vi "Adjust Graph.vi"(7 "log?":bool, 8 "error in (no error)":errorcluster, 9 "Secondary Graph":refnum<vi>, 10 "Primary Graph":refnum<vi>, 11 "Scan Driver.lvclass":refnum<class "Scan Driver.lvclass">) -> (0 "error out":errorcluster, 2 "High":dbl, 3 "Scan Driver.lvclass out":refnum<class "Scan Driver.lvclass">)   [LabVIEW 2015, in "Scan Driver.lvclass"]
uses:
  Scan Driver.lvclass
  Scan Driver.lvclass/Scan Driver.ctl
  Scanners/Scanner/Scanner.lvclass
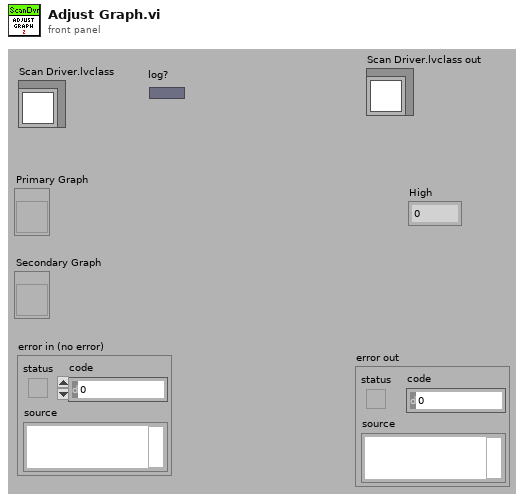
[diagram p1: front panel]
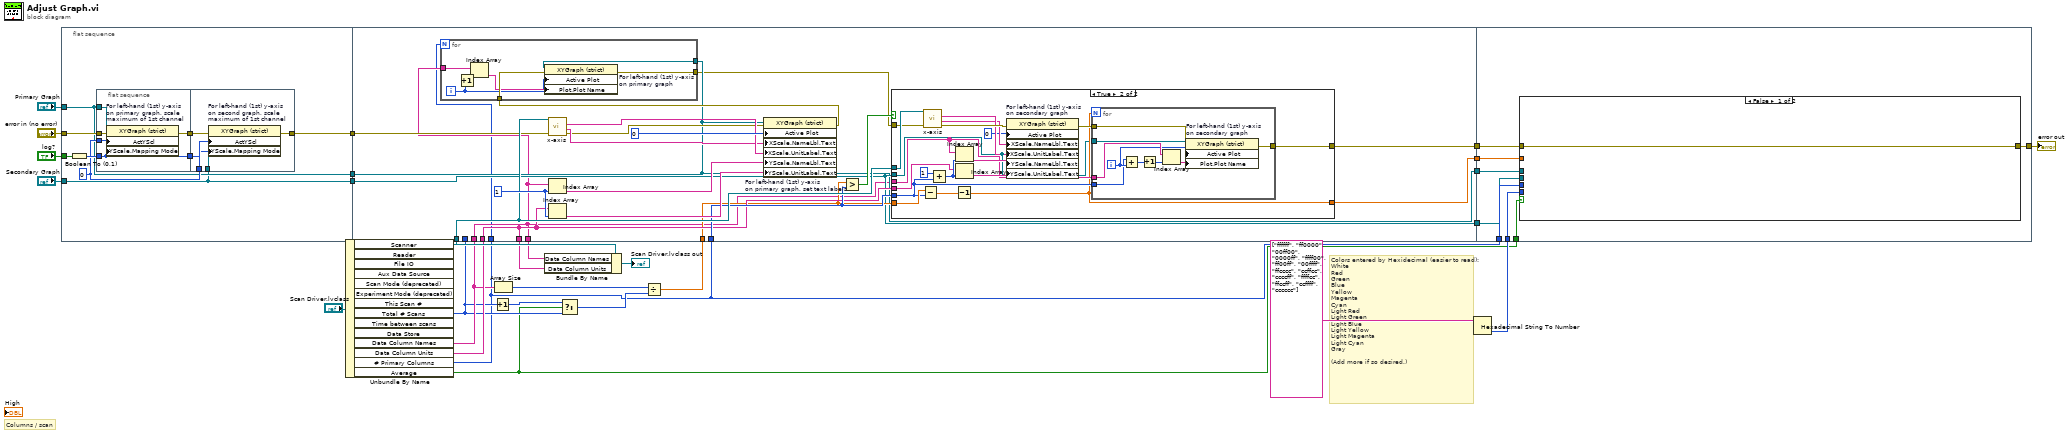
[diagram p0: block diagram]
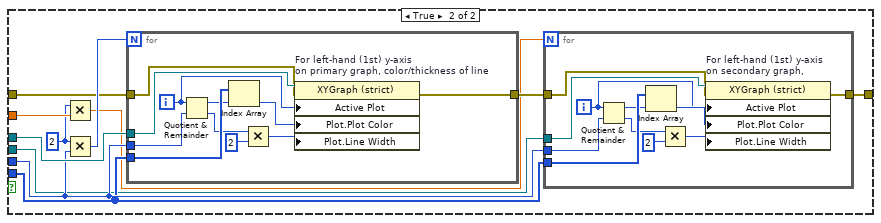
[diagram p3: hidden frame]
diagram:
  # "Columns / scan"
  # "Colors entered by Hexidecimal (easier to read):\nWhite\nRed\nGreen\nBlue\nYellow\nMagenta\nCyan\nLight Red\nLight Green\nLight Blue\nLight Yellow\nLight Magenta\nLight Cyan\nGray\n\n(Add more if so desired.)"
  n1 = flat-sequence {
    tunnel: "log?" -> [w37]
    tunnel: "Primary Graph" -> [w30]
    tunnel: "Secondary Graph" -> [w29]
    tunnel: "error in (no error)" -> [w35]
    tunnel: [w31] -> w17
    tunnel: [w30] -> w16
    tunnel: [w29] -> w15
    tunnel: w17 -> [w60]
    tunnel: w9 -> [w50]
    tunnel: w10 -> [w57]
    tunnel: w7 -> [w56]
    tunnel: [w50] -> w23
    tunnel: [w57] -> w22
    tunnel: w4 -> [_]
    tunnel: w16 -> [w51]
    tunnel: w3 -> [w61]
    tunnel: w15 -> [w53]
    tunnel: w1 -> [w58]
    tunnel: [w55] -> w14
    tunnel: [w51] -> w13
    tunnel: [w54] -> w12
    tunnel: [w53] -> w11
    tunnel: w1 -> [w48]
    tunnel: w14 -> [w111]
    tunnel: w2 -> [w112]
    tunnel: w20 -> [w110]
    tunnel: w13 -> [w109]
    tunnel: w1 -> [w108]
    tunnel: w12 -> [w107]
    tunnel: w11 -> [w106]
    tunnel: [w105] -> w18
    frame #0 {
      w33 = 0
      n2 = Boolean To (0,1)(Boolean=w37) -> (0, 1=w36:i16)
      n3 = flat-sequence {
        tunnel: w30 -> [w42]
        tunnel: w33 -> [w41]
        tunnel: w36 -> [w38]
        tunnel: w35 -> [w40]
        tunnel: [w39] -> w34
        tunnel: [w38] -> w32
        tunnel: w29 -> [w47]
        tunnel: w34 -> [w46]
        tunnel: w33 -> [w45]
        tunnel: w32 -> [w44]
        tunnel: [w43] -> w31
        frame #0 {
          n4 = property on="For left-hand (1st) y-axis\non primary graph, scale\nmaximum of 1st channel" class="XYGraph (strict)"(reference=w42, error in=w40, "ActYScl"=w41, "YScale.Mapping Mode"=w38) -> (error out=w39:errorcluster)  [unwired: 1 out]
        }
        frame #1 {
          n5 = property on="For left-hand (1st) y-axis\non second graph, scale\nmaximum of 1st channel" class="XYGraph (strict)"(reference=w47, error in=w46, "ActYScl"=w45, "YScale.Mapping Mode"=w44) -> (error out=w43:errorcluster)  [unwired: 1 out]
        }
      }
    }
    frame #1 {
      w65 = 1
      n6 = call-dynamic "x-axis.vi"("error in (no error)"=w60, "Scanner in"=w61) -> ("error out"=w59:errorcluster, "Label"=w66:string, "Unit"=w67:string)  [unwired: 6 in, 1 out]
      n7 = Index Array(array=w50, index=w65) -> (element=w64:string)
      n8 = Index Array(array=w57, index=w65) -> (element=w63:string)
      n9 = property on="For left-hand (1st) y-axis\non primary graph, set text labels" class="XYGraph (strict)"(reference=w51, error in=w59, "Active Plot"=0, "XScale.NameLbl.Text"=w66, "XScale.UnitLabel.Text"=w67, "YScale.NameLbl.Text"=w64, "YScale.UnitLabel.Text"=w63) -> (error out=w52:errorcluster)  [unwired: 1 out]
      n10 = for {
        N: w48 -> [_]
        tunnel: w52 -> [w75]
        tunnel: w51 -> [w74]
        tunnel: w50 -> [w73]
        tunnel: [w72] -> w49
        i -> [w70]
        n11 = Increment(x=w70) -> (x+1=w69:i32)
        n12 = Index Array(array=w73, index=w69) -> (element=w71:string)
        n13 = property on="For left-hand (1st) y-axis\non primary graph" class="XYGraph (strict)"(reference=w74, error in=w75, "Active Plot"=w70, "Plot.Plot Name"=w71) -> (error out=w72:errorcluster)  [unwired: 1 out]
      }
      n14 = Greater?(x=w56, y=w58) -> (0:w62:bool)
      n15 = case shown="True" w62 {
        tunnel: w53 -> [_ w77]
        tunnel: w49 -> [w76 w94]
        tunnel: w61 -> [_ w95]
        tunnel: w58 -> [_ w79]
        tunnel: w50 -> [_ w82]
        tunnel: w57 -> [_ w86]
        tunnel: w56 -> [_ w84]
        tunnel: [w76 w80] -> w55
        tunnel: [_ w78] -> w54
        frame False {
        }
        frame True {
          n16 = Subtract(x=w84, y=w79) -> (x-y=w83:dbl)
          n17 = call-dynamic "x-axis.vi"("error in (no error)"=w94, "Scanner in"=w95) -> ("error out"=w93:errorcluster, "Label"=w91:string, "Unit"=w92:string)  [unwired: 6 in, 1 out]
          n18 = Add(x=1, y=w79) -> (x+y=w89:u32)
          n19 = Decrement(x=w83) -> (x-1=w78:dbl)
          n20 = Index Array(array=w82, index=w89) -> (element=w85:string)
          n21 = Index Array(array=w86, index=w89) -> (element=w88:string)
          n22 = property on="For left-hand (1st) y-axis\non secondary graph" class="XYGraph (strict)"(reference=w77, error in=w93, "Active Plot"=0, "XScale.NameLbl.Text"=w91, "XScale.UnitLabel.Text"=w92, "YScale.NameLbl.Text"=w85, "YScale.UnitLabel.Text"=w88) -> (error out=w81:errorcluster)  [unwired: 1 out]
          n23 = for {
            N: w78 -> [_]
            tunnel: w82 -> [w101]
            tunnel: w77 -> [w104]
            tunnel: w81 -> [w103]
            tunnel: [w102] -> w80
            tunnel: w79 -> [w98]
            i -> [w100]
            n24 = Add(x=w98, y=w100) -> (x+y=w99:u32)
            n25 = Increment(x=w99) -> (x+1=w96:u32)
            n26 = Index Array(array=w101, index=w96) -> (element=w97:string)
            n27 = property on="For left-hand (1st) y-axis\non secondary graph" class="XYGraph (strict)"(reference=w104, error in=w103, "Active Plot"=w100, "Plot.Plot Name"=w97) -> (error out=w102:errorcluster)  [unwired: 1 out]
          }
        }
      }
    }
    frame #2 {
      n28 = case shown="False" w112 {
        tunnel: w111 -> [w113 w123]
        tunnel: w110 -> [_ w119]
        tunnel: w109 -> [_ w122]
        tunnel: w108 -> [_ w120]
        tunnel: w107 -> [_ w121]
        tunnel: w106 -> [_ w118]
        tunnel: [w113 w114] -> w105
        frame False {
        }
        frame True {
          w115 = 2
          n29 = Multiply(x=w115, y=w121) -> (x*y=w116:dbl)
          n30 = Multiply(x=w115, y=w120) -> (x*y=w124:u32)
          n31 = for {
            N: w124 -> [_]
            tunnel: w119 -> [w146]
            tunnel: w120 -> [w143]
            tunnel: w122 -> [w138]
            tunnel: w123 -> [w137]
            tunnel: [w136] -> w117
            i -> [w144]
            n32 = Quotient & Remainder(x=w144, y=w143) -> (x-y*floor(x/y)=w139:u32, floor(x/y)=w142:u32)
            n33 = Index Array(array=w146, index=w139) -> (element=w145:u32)
            n34 = Multiply(x=w142, y=2) -> (x*y=w141:u32)
            n35 = property on="For left-hand (1st) y-axis\non primary graph, color/thickness of line" class="XYGraph (strict)"(reference=w138, error in=w137, "Active Plot"=w144, "Plot.Plot Color"=w145, "Plot.Line Width"=w141) -> (error out=w136:errorcluster)  [unwired: 1 out]
          }
          n36 = for {
            N: w116 -> [_]
            tunnel: w120 -> [w125]
            tunnel: w119 -> [w135]
            tunnel: w118 -> [w134]
            tunnel: w117 -> [w133]
            tunnel: [w126] -> w114
            i -> [w130]
            n37 = Quotient & Remainder(x=w130, y=w125) -> (x-y*floor(x/y)=w131:u32, floor(x/y)=w129:u32)
            n38 = Index Array(array=w135, index=w131) -> (element=w132:u32)
            n39 = Multiply(x=w129, y=2) -> (x*y=w127:u32)
            n40 = property on="For left-hand (1st) y-axis\non secondary graph," class="XYGraph (strict)"(reference=w134, error in=w133, "Active Plot"=w130, "Plot.Plot Color"=w132, "Plot.Line Width"=w127) -> (error out=w126:errorcluster)  [unwired: 1 out]
          }
        }
      }
    }
  }
  n41 = Unbundle By Name("Scan Driver.lvclass") -> ("Scanner"=w3:refnum<class "Scanner.lvclass">, "Total # Scans"=w4:u32, "Data Column Names"=w9:string[], "Data Column Units"=w10:string[], "# Primary Columns"=w1:u32, "Average"=w2:bool)  [unwired: 8 out]
  n42 = Increment(x=w4) -> (x+1=w5:u32)
  n43 = Array Size(array=w9) -> (size(s)=w8:i32)
  n44 = Bundle By Name(cluster="Scan Driver.lvclass", "Data Column Names"=w23, "Data Column Units"=w22) -> (→"Scan Driver.lvclass out":refnum<class "Scan Driver.lvclass">)
  n45 = Select(t=w5, s=w2, f=w4) -> (s? t:f=w6:u32)
  n46 = Divide(x=w8, y=w6) -> (x/y=w7:dbl)
  n47 = Hexadecimal String To Number(string=string[] ["ffffff", "ff0000", "00ff00", "0000ff", "ffff00", "ff00ff", "00ffff", "ffcccc", "ccffcc", "ccccff", "ffffcc", "ffccff", "ccffff", "cccccc"]) -> (number=w20:u32[])  [unwired: 2 in, 1 out]
  "error out" <- w18
